vi "SuperAuton-CanBackAndForth.vi"(8 "error in (no error)":errorcluster, 9 "TimeToPull":dbl, 11 "Auton Event Queue Data":refnum<queue>) -> (0 "error out":errorcluster, 2 "Success?":bool, 3 "Auton Event Queue Data 2":refnum<queue>)   [LabVIEW 2014]
uses:
  Robot Global Data.vi
  <vilib>/Rock Robotics/WPI/RobotDrive/WPI_RobotDriveGetSetRefNum.vi
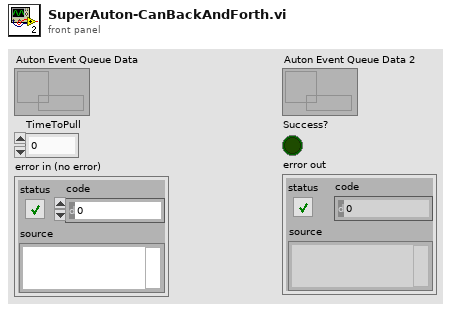
[diagram p1: front panel]
types:
  T1 = typedef "WPI_RobotDriveDevRef.ctl" = cluster{"DevStatus":errorcluster, "Motors[]":T2[], "Square Inputs":bool, "Max Output":dbl}
  T2 = typedef "WPI_MotorControlDeviceRef.ctl" = cluster{"DeviceStatus":errorcluster, "Type":T3, "PWM":cluster{"Controller":T4, "PWM Channel":T5, "DeadBand":T6}, "CAN":cluster{"Device Number":u8, "Control Mode":T7, "Semaphore":T8, "Max Vout":dbl, "TalonSRX Control Mode":T9}, "Invert":bool, "TransformRef":T10, "InvTransformRef":T10}
  T3 = typedef "WPI_MotorControlType.ctl" = enum16{"PWM", "CAN", "CANTalonSRX"}
  T4 = typedef "FPGA_TypedefDigitalModule.ctl" = enum16{"Controller 1"}
  T5 = typedef "FPGA_DIOPWMChannel.ctl" = enum8{"PWM 0", "PWM 1", "PWM 2", "PWM 3", "PWM 4", "PWM 5", "PWM 6", "PWM 7", "PWM 8", "PWM 9", "PWM MXP 0", "PWM MXP 1", "PWM MXP 2", "PWM MXP 3", "PWM MXP 4", "PWM MXP 5", "PWM MXP 6", "PWM MXP 7", "PWM MXP 8", "PWM MXP 9", "Invalid"}
  T6 = typedef "WPI_PWMDeadband.ctl" = cluster{"Name":string, "maxPositivePwm":i32, "minPositivePwm":i32, "centerPwm":i32, "maxNegativePwm":i32, "minNegativePwm":i32, "angularRange":u16}
  T7 = typedef "WPI_CANJaguar_ControlMode.ctl" = enum8{"Percent VBus", "Current", "Speed", "Position", "Voltage"}
  T8 = typedef "Semaphore RefNum" = refnum<k1>
  T9 = typedef "WPI_CANTalonSRX_APIControlMode.ctl" = enum8{"Percent VBus", "Speed", "Position", "Slave", "Unchanged / Invalid"}
  T10 = typedef "WPI_PWMTransform_ConPane.ctl" = refnum<vi>
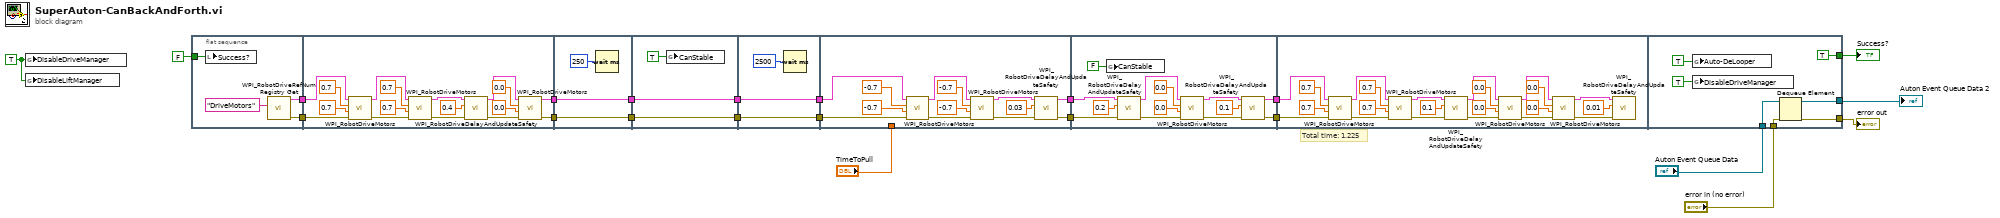
[diagram p0: block diagram]
diagram:
  w18 = TRUE ("Success?")
  # "Total time: 1.225"
  n1 = global write "Robot Global Data.vi" "DisableDriveManager"(w18) -> ()
  n2 = global write "Robot Global Data.vi" "DisableLiftManager"(w18) -> ()
  n3 = flat-sequence {
    tunnel: FALSE ("Success?") -> [w26]
    tunnel: [w24] -> w16
    tunnel: [w23] -> w17
    tunnel: w17 -> [w29]
    tunnel: w16 -> [w30]
    tunnel: [w43] -> w15
    tunnel: [w42] -> w14
    tunnel: w15 -> [w46]
    tunnel: [w46] -> w13
    tunnel: w14 -> [w45]
    tunnel: [w45] -> w12
    tunnel: w13 -> [w48]
    tunnel: w12 -> [w47]
    tunnel: [w48] -> w11
    tunnel: [w47] -> w10
    tunnel: [w51] -> w9
    tunnel: w11 -> [w51]
    tunnel: [w50] -> w8
    tunnel: w10 -> [w50]
    tunnel: "TimeToPull" -> [_]
    tunnel: w9 -> [w56]
    tunnel: w8 -> [w54]
    tunnel: [w60] -> w7
    tunnel: [w59] -> w6
    tunnel: w7 -> [w72]
    tunnel: w6 -> [w69]
    tunnel: [w67] -> w2
    tunnel: [w66] -> w1
    tunnel: w2 -> [w91]
    tunnel: w1 -> [w90]
    tunnel: [TRUE ("Success?")] -> w5
    tunnel: "Auton Event Queue Data" -> [w104]
    tunnel: "error in (no error)" -> [w103]
    tunnel: [w102] -> w20
    tunnel: [w101] -> w19
    frame #0 {
      n4 = local write "Success?"(w26) -> ()
      n5 = call <vilib>:"WPI_RobotDriveRefNum Registry Get.vi"("refnum name"="DriveMotors") -> ("error out"=w23:errorcluster, "RobotDriveDevRef"=w24:T1)  [unwired: 9 in]
    }
    frame #1 {
      n6 = call <vilib>:"WPI_RobotDriveMotors.vi"("error in (no error)"=w29, "RightSpeed"=0.7 ("Y axis value"), "LeftSpeed"=0.7 ("X axis value"), "RobotDriveDevRef"=w30) -> ("error out"=w27:errorcluster, "RobotDriveDevRef"=w28:T1)  [unwired: 5 in, 1 out]
      n7 = call <vilib>:"WPI_RobotDriveMotors.vi"("error in (no error)"=w27, "RightSpeed"=0.7 ("Y axis value"), "LeftSpeed"=0.7 ("X axis value"), "RobotDriveDevRef"=w28) -> ("error out"=w38:errorcluster, "RobotDriveDevRef"=w39:T1)  [unwired: 5 in, 1 out]
      n8 = call <vilib>:"WPI_RobotDriveDelayAndUpdateSafety.vi"("error in (no error)"=w38, "Delay (s)"=0.4, "RobotDriveDevRef"=w39) -> ("error out"=w35:errorcluster, "RobotDriveDevRef 2"=w36:T1)  [unwired: 7 in]
      n9 = call <vilib>:"WPI_RobotDriveMotors.vi"("error in (no error)"=w35, "RightSpeed"=0.0 ("Y axis value"), "LeftSpeed"=0.0 ("X axis value"), "RobotDriveDevRef"=w36) -> ("error out"=w42:errorcluster, "RobotDriveDevRef"=w43:T1)  [unwired: 5 in, 1 out]
    }
    frame #2 {
      n10 = Wait (ms)(milliseconds to wait=u32 250) -> ()  [unwired: 1 out]
    }
    frame #3 {
      n11 = global write "Robot Global Data.vi" "CanStable"(TRUE) -> ()
    }
    frame #4 {
      n12 = Wait (ms)(milliseconds to wait=u32 2500) -> ()  [unwired: 1 out]
    }
    frame #5 {
      n13 = call <vilib>:"WPI_RobotDriveMotors.vi"("error in (no error)"=w54, "RightSpeed"=-0.7 ("Y axis value"), "LeftSpeed"=-0.7 ("X axis value"), "RobotDriveDevRef"=w56) -> ("error out"=w53:errorcluster, "RobotDriveDevRef"=w55:T1)  [unwired: 5 in, 1 out]
      n14 = call <vilib>:"WPI_RobotDriveMotors.vi"("error in (no error)"=w53, "RightSpeed"=-0.7 ("Y axis value"), "LeftSpeed"=-0.7 ("X axis value"), "RobotDriveDevRef"=w55) -> ("error out"=w62:errorcluster, "RobotDriveDevRef"=w63:T1)  [unwired: 5 in, 1 out]
      n15 = call <vilib>:"WPI_RobotDriveDelayAndUpdateSafety.vi"("error in (no error)"=w62, "Delay (s)"=0.03, "RobotDriveDevRef"=w63) -> ("error out"=w59:errorcluster, "RobotDriveDevRef 2"=w60:T1)  [unwired: 7 in]
    }
    frame #6 {
      n16 = global write "Robot Global Data.vi" "CanStable"(FALSE) -> ()
      n17 = call <vilib>:"WPI_RobotDriveDelayAndUpdateSafety.vi"("error in (no error)"=w69, "Delay (s)"=0.2, "RobotDriveDevRef"=w72) -> ("error out"=w70:errorcluster, "RobotDriveDevRef 2"=w71:T1)  [unwired: 7 in]
      n18 = call <vilib>:"WPI_RobotDriveMotors.vi"("error in (no error)"=w70, "RightSpeed"=0.0 ("Y axis value"), "LeftSpeed"=0.0 ("X axis value"), "RobotDriveDevRef"=w71) -> ("error out"=w76:errorcluster, "RobotDriveDevRef"=w77:T1)  [unwired: 5 in, 1 out]
      n19 = call <vilib>:"WPI_RobotDriveDelayAndUpdateSafety.vi"("error in (no error)"=w76, "Delay (s)"=0.1, "RobotDriveDevRef"=w77) -> ("error out"=w66:errorcluster, "RobotDriveDevRef 2"=w67:T1)  [unwired: 7 in]
    }
    frame #7 {
      n20 = call <vilib>:"WPI_RobotDriveMotors.vi"("error in (no error)"=w90, "RightSpeed"=0.7 ("Y axis value"), "LeftSpeed"=0.7 ("X axis value"), "RobotDriveDevRef"=w91) -> ("error out"=w92:errorcluster, "RobotDriveDevRef"=w93:T1)  [unwired: 5 in, 1 out]
      n21 = call <vilib>:"WPI_RobotDriveMotors.vi"("error in (no error)"=w92, "RightSpeed"=0.7 ("Y axis value"), "LeftSpeed"=0.7 ("X axis value"), "RobotDriveDevRef"=w93) -> ("error out"=w97:errorcluster, "RobotDriveDevRef"=w98:T1)  [unwired: 5 in, 1 out]
      n22 = call <vilib>:"WPI_RobotDriveDelayAndUpdateSafety.vi"("error in (no error)"=w97, "Delay (s)"=0.1, "RobotDriveDevRef"=w98) -> ("error out"=w81:errorcluster, "RobotDriveDevRef 2"=w82:T1)  [unwired: 7 in]
      n23 = call <vilib>:"WPI_RobotDriveMotors.vi"("error in (no error)"=w81, "RightSpeed"=0.0 ("Y axis value"), "LeftSpeed"=0.0 ("X axis value"), "RobotDriveDevRef"=w82) -> ("error out"=w80:errorcluster, "RobotDriveDevRef"=w79:T1)  [unwired: 5 in, 1 out]
      n24 = call <vilib>:"WPI_RobotDriveMotors.vi"("error in (no error)"=w80, "RightSpeed"=0.0 ("Y axis value"), "LeftSpeed"=0.0 ("X axis value"), "RobotDriveDevRef"=w79) -> ("error out"=w87:errorcluster, "RobotDriveDevRef"=w88:T1)  [unwired: 5 in, 1 out]
      n25 = call <vilib>:"WPI_RobotDriveDelayAndUpdateSafety.vi"("error in (no error)"=w87, "Delay (s)"=0.01, "RobotDriveDevRef"=w88) -> ()  [unwired: 7 in, 2 out]
    }
    frame #8 {
      n26 = global write "Robot Global Data.vi" "Auto-DeLooper"(TRUE ("DisableDriveManager")) -> ()
      n27 = global write "Robot Global Data.vi" "DisableDriveManager"(TRUE ("DisableDriveManager")) -> ()
      n28 = Dequeue Element(queue=w104, error in (no error)=w103) -> (queue out=w102:refnum<queue>, error out=w101:errorcluster)  [unwired: 1 in, 2 out]
    }
  }
  "error out" <- w19
  "Auton Event Queue Data 2" <- w20
  "Success?" <- w5
